vi "Q-3.vi"(11 "Error_In":errorcluster) -> (4 "Place_Option_Out":string, 15 "Error_Out":errorcluster)   [LabVIEW 2023]
uses:
  Controls/Place_Option.ctl
panel:
  in  "Place_Option":T1
  # "Do you like \n‘sea’, ‘ocean’, ‘mountains"
  # "Excellent choice! Now, to further refine the magic that will reveal your destiny, I must ask you one more question"
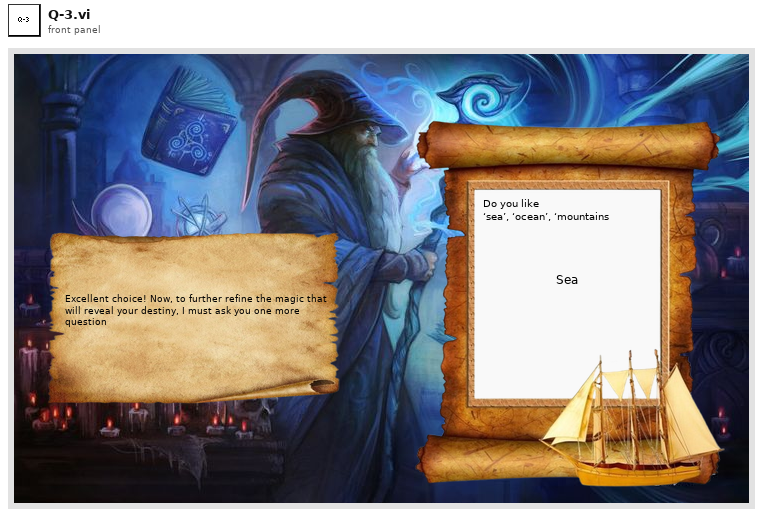
[diagram p1: front panel]
types:
  T1 = typedef "Place_Option.ctl" = enum16{"Sea", "Ocean", "Mountain"}
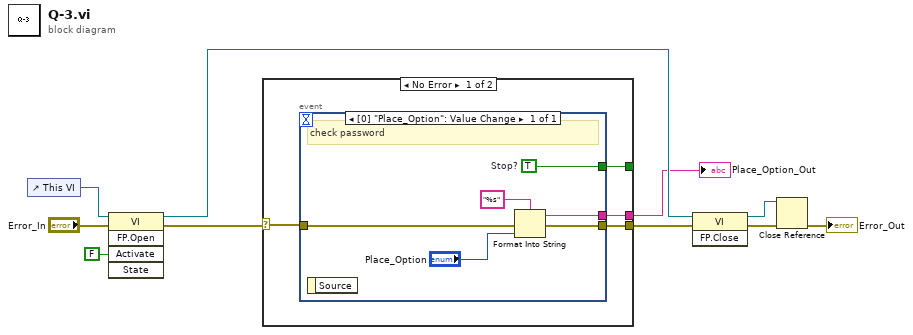
[diagram p0: block diagram]
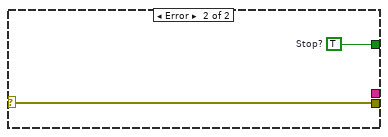
[diagram p2: hidden frame]
diagram:
  n1 = control-ref of="This VI"() -> (w7:refnum<vi>)
  n2 = invoke class="VI" method="FP.Open"(reference=w7, error in="Error_In", "Activate"=FALSE ("Activate?")) -> (reference out=w4:refnum<vi>, error out=w8:errorcluster)  [unwired: 2 in, 3 out]
  n3 = case shown="No Error" w8 {
    selector: w8 -> [w14 w22]
    tunnel: [w13 w22] -> w9
    tunnel: [w12 w21] -> _
    tunnel: [w11 _] -> w1
    frame No Error {
      n4 = event shown="[0] \"Place_Option\": Value Change" {
        selector: _ -> [_]
        dyn-events: _ -> [_]
        timeout: _ -> [_]
        tunnel: w14 -> [w18]
        tunnel: [w17] -> w13
        tunnel: [w20] -> w12
        tunnel: [w15] -> w11
        event Value Change {
          w20 = TRUE  # Stop?
          # "check password"
          n5 = event-data() -> ()  [unwired: 1 in, 1 out]
          n6 = Format Into String(format string="%s", error in=w18, "Place_Option") -> (resulting string=w15:string, error out=w17:errorcluster)  [unwired: 1 in]
        }
      }
    }
    frame Error {
      w21 = TRUE  # Stop?
    }
  }
  "Place_Option_Out" <- w1
  n7 = invoke class="VI" method="FP.Close"(reference=w4, error in=w9) -> (reference out=w2:refnum<vi>, error out=w5:errorcluster)  [unwired: 1 in, 1 out]
  n8 = Close Reference(reference=w2, error in (no error)=w5) -> (error out=→"Error_Out":errorcluster)
